vi "PB_Cburn_hold.vi"(11 "Optimize active channels":bool[](array[boolean])=[FALSE, FALSE, FALSE, TRUE]) -> (2 "Return":i32, 3 "String":string)   [LabVIEW 2012]
uses:
  Channels.vi
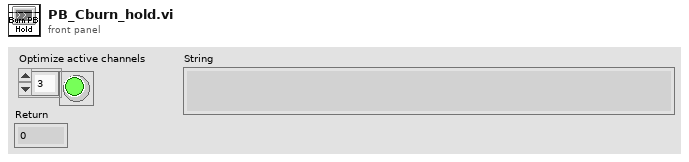
[diagram p1: front panel]
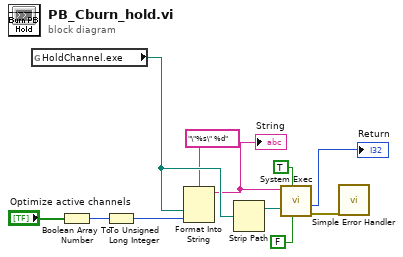
[diagram p0: block diagram]
diagram:
  n1 = global read "Channels.vi" "HoldChannel.exe"() -> (w10:path)
  n2 = Boolean Array To Number(Boolean array="Optimize active channels") -> (number=w6:u32)
  n3 = To Unsigned Long Integer(number=w6) -> (unsigned 32bit integer=w11:u32)
  n4 = Format Into String(format string="\"%s\" %d", w10, w11) -> (resulting string=w8:string)  [unwired: 2 in, 1 out]
  "String" <- w8
  n5 = Strip Path(path=w10) -> (stripped path=w2:path)  [unwired: 1 out]
  n6 = call <vilib>:"System Exec.vi"("run minimized? (F)"=FALSE ("Wait until done"), "wait until completion? (T)"=TRUE ("Wait until done"), "working directory"=w2, "command line"=w8) -> ("error out"=w9:errorcluster, "return code"=→"Return":i32)  [unwired: 4 in, 2 out]
  n7 = call <vilib>:"Simple Error Handler.vi"("error in (no error)"=w9) -> ()  [unwired: 4 in, 5 out]
